vi "Interger Range Case Structure.vi"() -> ()   [LabVIEW 2020]
panel:
  in  "Numeric":dbl
  # "Interger Ranges Case Structure"
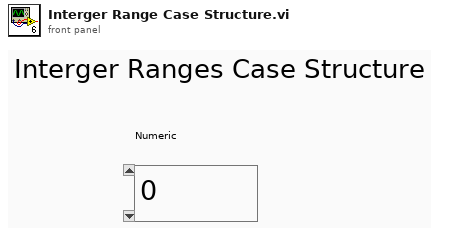
[diagram p1: front panel]
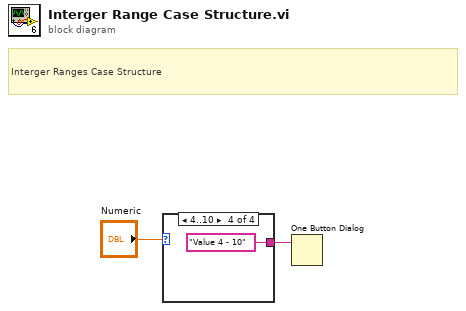
[diagram p0: block diagram]
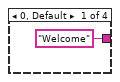
[diagram p2: hidden frame]
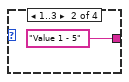
[diagram p3: hidden frame]
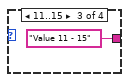
[diagram p4: hidden frame]
diagram:
  # "Interger Ranges Case Structure"
  n1 = case shown="4..10" "Numeric" {
    tunnel: ["Welcome" "Value 1 - 5" "Value 11 - 15" "Value 4 - 10"] -> w1
    frame 0, Default {
    }
    frame 1..3 {
    }
    frame 11..15 {
    }
    frame 4..10 {
    }
  }
  n2 = One Button Dialog(message=w1) -> ()  [unwired: 1 in, 1 out]
